vi "EXEvi.vi"() -> ()   [LabVIEW 2019]
panel:
  out "Waveform Chart":dbl(graph)
  in  "Read File":bool=TRUE
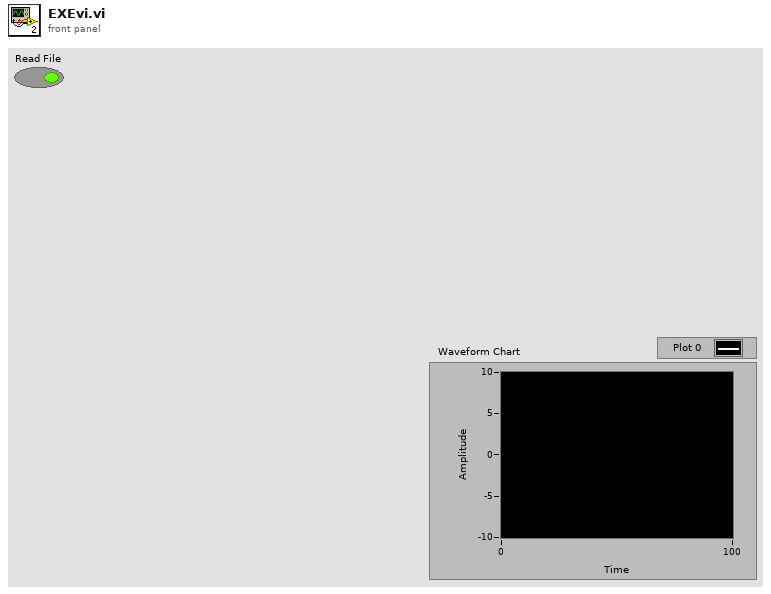
[diagram p1: front panel]
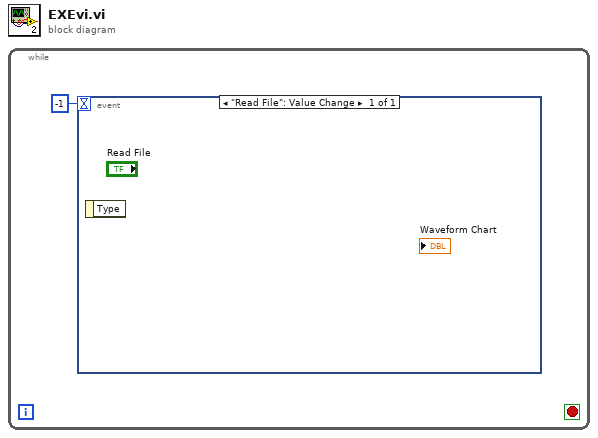
[diagram p0: block diagram]
diagram:
  n1 = while {
    stop <- _ stop-if-true
    n2 = event shown="[0] \"Read File\": Value Change" {
      selector: _ -> [_]
      dyn-events: _ -> [_]
      timeout: -1 -> [_]
      event "Read File": Value Change {
        n3 = event-data() -> ()  [unwired: 1 in, 1 out]
      }
    }
  }
